vi "Main.vi"() -> ()   [LabVIEW 2014]
uses:
  <vilib>/myRIO/Common/Instrument Driver Framework/myRIO v1.0/PWM/vis/myRIO v1.1 Open PWM.vi
  <vilib>/myRIO/Common/Instrument Driver Framework/myRIO v1.0/PWM/vis/myRIO v1.2 Open PWM.vi
  <vilib>/myRIO/Common/Instrument Driver Framework/myRIO v1.0/UART/vis/myRIO v1.0 Close UART.vi
  <vilib>/myRIO/Common/Instrument Driver Framework/Utilities/vis/Validate Channels.vi
  <vilib>/myRIO/Common/Instrument Driver Framework/myRIO v1.0/PWM/vis/myRIO v1.0 Reserve PWM.vi
  <vilib>/myRIO/Common/Instrument Driver Framework/myRIO v1.0/PWM/vis/myRIO v1.0 Build MUX Configuration PWM.vi
  <vilib>/myRIO/Common/Instrument Driver Framework/myRIO v1.0/Resource Manager/vis/myRIO v1.0 Reserve Channel List.vi
  <vilib>/myRIO/Common/Instrument Driver Framework/myRIO v1.0/Resource Manager/vis/myRIO v1.0 Create Configuration List.vi
  <vilib>/myRIO/Common/Instrument Driver Framework/myRIO v1.0/Resource Manager/vis/myRIO v1.0 Reserve Channel.vi
  <vilib>/myRIO/Common/Instrument Driver Framework/myRIO v1.0/Resource Manager/vis/myRIO v1.0 Unreserve Channel.vi
  <vilib>/myRIO/Common/Instrument Driver Framework/myRIO v1.0/Resource Manager/vis/myRIO v1.0 Build Mutex Name.vi
  <vilib>/myRIO/Common/Instrument Driver Framework/Utilities/vis/Set_Get Target Info.vi
  <vilib>/Utility/error.llb/Error Cluster From Error Code.vi
  <vilib>/Utility/VariantDataType/GetNumericInfo.vi
  <vilib>/myRIO/Common/Instrument Driver Framework/myRIO v1.0/myRIO v1.1 Open.vi
  <vilib>/myRIO/Common/Instrument Driver Framework/Utilities/vis/IO Manager.vi
  <vilib>/myRIO/Common/Instrument Driver Framework/Utilities/vis/Configuration Manager.vi
  <vilib>/myRIO/Common/Instrument Driver Framework/myRIO v1.0/Resource Manager/vis/myRIO v1.0 Configure IO.vi
  <vilib>/myRIO/Common/Instrument Driver Framework/myRIO v1.0/myRIO v1.0 Close.vi
  <vilib>/myRIO/Common/Instrument Driver Framework/myRIO v1.0/myRIO v1.2 Open.vi
  <vilib>/myRIO/Common/Instrument Driver Framework/myRIO v1.0/PWM/vis/myRIO v1.0 Write PWM.vi
  <vilib>/myRIO/Common/Instrument Driver Framework/Utilities/vis/FPGA Ref Manager.vi
  <vilib>/myRIO/Common/Instrument Driver Framework/myRIO v1.0/myRIO v1.0 Reset FPGA.vi
  <vilib>/myRIO/Common/Instrument Driver Framework/myRIO v1.0/IRQ/vis/myRIO v1.0 IRQ Info FGV.vi
  <vilib>/myRIO/Common/Instrument Driver Framework/myRIO v1.0/IRQ/vis/myRIO v1.0 Timer IRQ Info FGV.vi
  <vilib>/myRIO/Common/Instrument Driver Framework/myRIO v1.0/IRQ/vis/myRIO v1.0 ISR Agent.vi
  <vilib>/myRIO/Instrument Drivers/Utilities/Utilities.lvlib
  <vilib>/myRIO/Instrument Drivers/Onboard IO/PWM/PWM.lvlib
panel:
  in  "freq [Hz] 9":dbl=50.0
  out "duty cycle [%] 9":dbl
  out "pulse width [ms] 9":dbl=1.5
  out "offset [%FS] 7":dbl
  in  "null offset 7":bool
  in  "freq [Hz] 6":dbl=50.0
  in  "null offset 6":bool
  in  "position [%FS] 6":dbl(slide) scale=-200.0..200.0
  out "duty cycle [%] 6":dbl
  out "pulse width [ms] 6":dbl=1.5
  out "offset [%FS] 6":dbl
  in  "freq [Hz] 5":dbl=50.0
  in  "null offset 5":bool
  in  "position [%FS] 5":dbl(slide) scale=-200.0..200.0
  out "duty cycle [%] 5":dbl
  out "pulse width [ms] 5":dbl=1.5
  out "offset [%FS] 5":dbl
  in  "position [%FS] 4":dbl(slide) scale=-200.0..200.0
  out "pulse width [ms] 3":dbl=1.5
  out "duty cycle [%] 3":dbl
  out "offset [%FS] 3":dbl
  in  "null offset 3":bool
  in  "freq [Hz] 3":dbl=50.0
  in  "position [%FS] 3":dbl(slide) scale=-200.0..200.0
  in  "freq [Hz] 2":dbl=50.0
  in  "null offset 2":bool
  in  "position [%FS] 2":dbl(slide) scale=-200.0..200.0
  out "duty cycle [%] 2":dbl
  out "pulse width [ms] 2":dbl=1.5
  out "offset [%FS] 2":dbl
  out "duty cycle [%]":dbl
  out "pulse width [ms]":dbl=1.5
  out "offset [%FS]":dbl
  in  "freq [Hz]":dbl=50.0
  in  "null offset":bool
  in  "position [%FS]":dbl(slide) scale=-200.0..200.0
  in  "[ESC]":bool
  # "Servo  3"
  # "Servo  1"
  # "Servo  2"
  # "Servo  6"
  # "Servo  5"
  # "Servo  4"
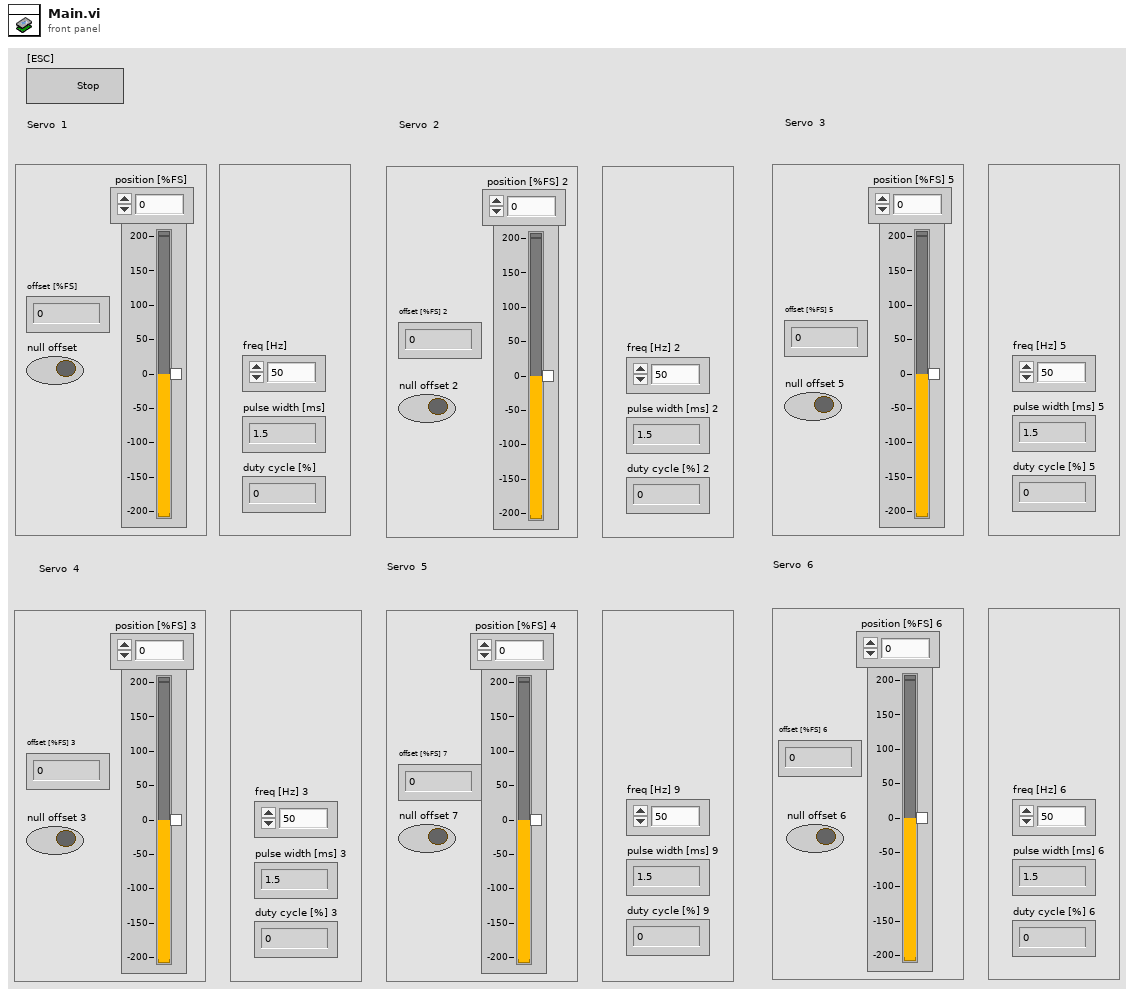
[diagram p1: front panel]
types:
  T1 = typedef "PWM.lvlib/PWM Reference.ctl" = cluster{"myRIO Reference":T2, "PWM Channels Enum":T6, "PWM Configuration":T7}
  T2 = typedef "myRIO Generic Hardware Reference.ctl" = cluster{"myRIO Model":T3, "myRIO Hardware Reference":T4}
  T3 = typedef "Hardware Version Enum.ctl" = enum16{"Unknown", "myRIO-1900", "myRIO-1950"}
  T4 = typedef "myRIO v1.0 Reference.ctl" = cluster{"Generic FPGA Reference":T5, "Allow multiple opens":bool}
  T5 = typedef "Generic FPGA Reference.ctl" = refnum<k20>
  T6 = typedef "PWM Channels Enum.ctl" = enum16{"Not Connected", "C/PWM0", "C/PWM1", "A/PWM0", "A/PWM1", "A/PWM2", "B/PWM0", "B/PWM1", "B/PWM2"}
  T7 = typedef "PWM.lvlib/PWM Configuration.ctl" = cluster{"Frequency":dbl, "Duty Cycle":dbl}
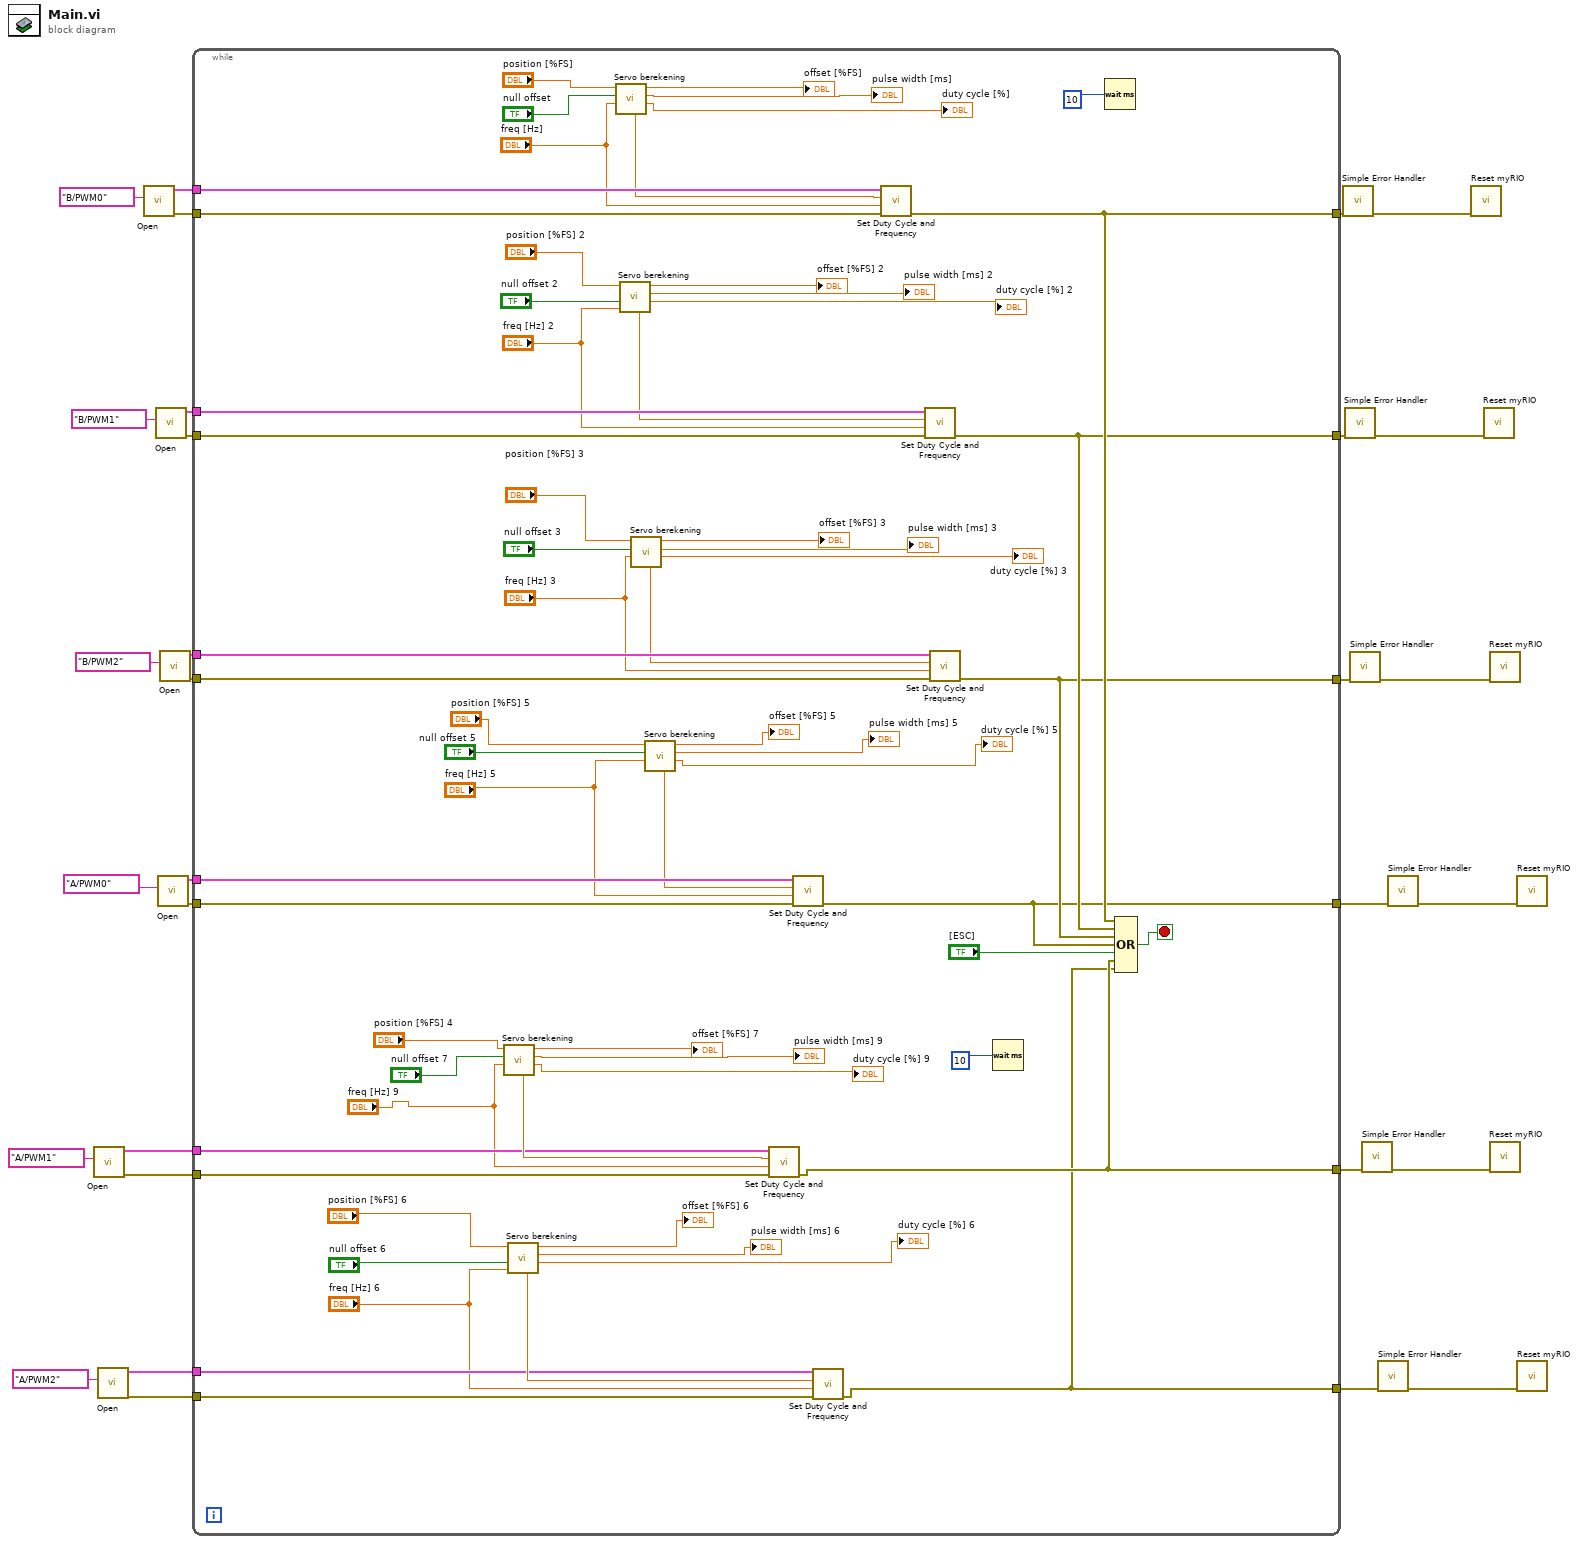
[diagram p0: block diagram]
diagram:
  n1 = call <vilib>:"Open.vi"("Channel Name"=tag "A/PWM1") -> ("error out"=w4:errorcluster, "PWM Ref Out"=w5:T1)  [unwired: 9 in]
  n2 = call <vilib>:"Open.vi"("Channel Name"=tag "A/PWM2") -> ("error out"=w1:errorcluster, "PWM Ref Out"=w2:T1)  [unwired: 9 in]
  n3 = call <vilib>:"Open.vi"("Channel Name"=tag "B/PWM0") -> ("error out"=w28:errorcluster, "PWM Ref Out"=w29:T1)  [unwired: 9 in]
  n4 = call <vilib>:"Open.vi"("Channel Name"=tag "B/PWM1") -> ("error out"=w25:errorcluster, "PWM Ref Out"=w24:T1)  [unwired: 9 in]
  n5 = call <vilib>:"Open.vi"("Channel Name"=tag "A/PWM0") -> ("error out"=w14:errorcluster, "PWM Ref Out"=w13:T1)  [unwired: 9 in]
  n6 = call <vilib>:"Open.vi"("Channel Name"=tag "B/PWM2") -> ("error out"=w23:errorcluster, "PWM Ref Out"=w22:T1)  [unwired: 9 in]
  n7 = while {
    tunnel: w29 -> [w93]
    tunnel: w28 -> [w92]
    tunnel: [w74] -> w27
    tunnel: w25 -> [w87]
    tunnel: w24 -> [w88]
    tunnel: w23 -> [w85]
    tunnel: w22 -> [w86]
    tunnel: [w73] -> w21
    tunnel: [w72] -> w20
    tunnel: w14 -> [w61]
    tunnel: w13 -> [w60]
    tunnel: [w59] -> w11
    tunnel: [w52] -> w9
    tunnel: [w51] -> w7
    tunnel: w5 -> [w50]
    tunnel: w4 -> [w49]
    tunnel: w2 -> [w48]
    tunnel: w1 -> [w47]
    stop <- w75 stop-if-true
    n8 = call "Servo berekening.vi"("freq [Hz]"="freq [Hz] 9", "null offset"="null offset 7", "position [%FS] in"="position [%FS] 4") -> ("Duty Cycle [%]"=→"duty cycle [%] 9":dbl, "Puls Width [ms]"=→"pulse width [ms] 9":dbl, "position [%FS] out"=→"offset [%FS] 7":dbl, "Duty Cycle"=w54:dbl)  [unwired: 5 in]
    n9 = call "Servo berekening.vi"("freq [Hz]"="freq [Hz] 6", "null offset"="null offset 6", "position [%FS] in"="position [%FS] 6") -> ("Duty Cycle [%]"=→"duty cycle [%] 6":dbl, "Puls Width [ms]"=→"pulse width [ms] 6":dbl, "position [%FS] out"=→"offset [%FS] 6":dbl, "Duty Cycle"=w53:dbl)  [unwired: 5 in]
    n10 = call "Servo berekening.vi"("freq [Hz]"="freq [Hz]", "null offset"="null offset", "position [%FS] in"="position [%FS]") -> ("Duty Cycle [%]"=→"duty cycle [%]":dbl, "Puls Width [ms]"=→"pulse width [ms]":dbl, "position [%FS] out"=→"offset [%FS]":dbl, "Duty Cycle"=w70:dbl)  [unwired: 5 in]
    n11 = call "Servo berekening.vi"("freq [Hz]"="freq [Hz] 2", "null offset"="null offset 2", "position [%FS] in"="position [%FS] 2") -> ("Duty Cycle [%]"=→"duty cycle [%] 2":dbl, "Puls Width [ms]"=→"pulse width [ms] 2":dbl, "position [%FS] out"=→"offset [%FS] 2":dbl, "Duty Cycle"=w69:dbl)  [unwired: 5 in]
    n12 = call "Servo berekening.vi"("freq [Hz]"="freq [Hz] 3", "null offset"="null offset 3", "position [%FS] in"="position [%FS] 3") -> ("Duty Cycle [%]"=→"duty cycle [%] 3":dbl, "Puls Width [ms]"=→"pulse width [ms] 3":dbl, "position [%FS] out"=→"offset [%FS] 3":dbl, "Duty Cycle"=w64:dbl)  [unwired: 5 in]
    n13 = call "Servo berekening.vi"("freq [Hz]"="freq [Hz] 5", "null offset"="null offset 5", "position [%FS] in"="position [%FS] 5") -> ("Duty Cycle [%]"=→"duty cycle [%] 5":dbl, "Puls Width [ms]"=→"pulse width [ms] 5":dbl, "position [%FS] out"=→"offset [%FS] 5":dbl, "Duty Cycle"=w58:dbl)  [unwired: 5 in]
    n14 = call <vilib>:"Set Duty Cycle and Frequency.vi"("error in (no error)"=w49, "Frequency [Hz]"="freq [Hz] 9", "Duty Cycle"=w54, "PWM Ref In"=w50) -> ("error out"=w52:errorcluster)  [unwired: 5 in, 1 out]
    n15 = call <vilib>:"Set Duty Cycle and Frequency.vi"("error in (no error)"=w61, "Frequency [Hz]"="freq [Hz] 5", "Duty Cycle"=w58, "PWM Ref In"=w60) -> ("error out"=w59:errorcluster)  [unwired: 5 in, 1 out]
    n16 = call <vilib>:"Set Duty Cycle and Frequency.vi"("error in (no error)"=w47, "Frequency [Hz]"="freq [Hz] 6", "Duty Cycle"=w53, "PWM Ref In"=w48) -> ("error out"=w51:errorcluster)  [unwired: 5 in, 1 out]
    n17 = call <vilib>:"Set Duty Cycle and Frequency.vi"("error in (no error)"=w92, "Frequency [Hz]"="freq [Hz]", "Duty Cycle"=w70, "PWM Ref In"=w93) -> ("error out"=w74:errorcluster)  [unwired: 5 in, 1 out]
    n18 = call <vilib>:"Set Duty Cycle and Frequency.vi"("error in (no error)"=w87, "Frequency [Hz]"="freq [Hz] 2", "Duty Cycle"=w69, "PWM Ref In"=w88) -> ("error out"=w73:errorcluster)  [unwired: 5 in, 1 out]
    n19 = call <vilib>:"Set Duty Cycle and Frequency.vi"("error in (no error)"=w85, "Frequency [Hz]"="freq [Hz] 3", "Duty Cycle"=w64, "PWM Ref In"=w86) -> ("error out"=w72:errorcluster)  [unwired: 5 in, 1 out]
    n20 = Wait (ms)(milliseconds to wait=u32 10) -> ()  [unwired: 1 out]
    n21 = Wait (ms)(milliseconds to wait=u32 10) -> ()  [unwired: 1 out]
    n22 = Compound Arithmetic op=OR(w74, w73, w72, w59, "[ESC]", w52, w51) -> (w75:bool)
  }
  n23 = call <vilib>:"Simple Error Handler.vi"("error in (no error)"=w27) -> ("error out"=w30:errorcluster)  [unwired: 4 in, 4 out]
  n24 = call <vilib>:"Simple Error Handler.vi"("error in (no error)"=w21) -> ("error out"=w19:errorcluster)  [unwired: 4 in, 4 out]
  n25 = call <vilib>:"Simple Error Handler.vi"("error in (no error)"=w20) -> ("error out"=w18:errorcluster)  [unwired: 4 in, 4 out]
  n26 = call <vilib>:"Simple Error Handler.vi"("error in (no error)"=w9) -> ("error out"=w10:errorcluster)  [unwired: 4 in, 4 out]
  n27 = call <vilib>:"Simple Error Handler.vi"("error in (no error)"=w7) -> ("error out"=w8:errorcluster)  [unwired: 4 in, 4 out]
  n28 = call <vilib>:"Simple Error Handler.vi"("error in (no error)"=w11) -> ("error out"=w26:errorcluster)  [unwired: 4 in, 4 out]
  n29 = call <vilib>:"Reset myRIO.vi"("error in (no error)"=w30) -> ()  [unwired: 10 in, 1 out]
  n30 = call <vilib>:"Reset myRIO.vi"("error in (no error)"=w19) -> ()  [unwired: 10 in, 1 out]
  n31 = call <vilib>:"Reset myRIO.vi"("error in (no error)"=w18) -> ()  [unwired: 10 in, 1 out]
  n32 = call <vilib>:"Reset myRIO.vi"("error in (no error)"=w10) -> ()  [unwired: 10 in, 1 out]
  n33 = call <vilib>:"Reset myRIO.vi"("error in (no error)"=w26) -> ()  [unwired: 10 in, 1 out]
  n34 = call <vilib>:"Reset myRIO.vi"("error in (no error)"=w8) -> ()  [unwired: 10 in, 1 out]
